vi "Freq elettrotest PS global.vi"() -> ()   [LabVIEW 2019]
panel:
  in  "Freq elettrotets PS":dbl
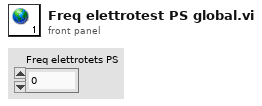
[diagram p1: front panel]
diagram:
